vi "LWXPS_PositionerCompensationDualLoopNotchFilterGet.vi"(0 "XPS Reference IN":refnum<k24>, 5 "Positioner Name":string, 7 "Notch Number":i32, 11 "LabVIEW error IN":errorcluster) -> (3 "XPS Reference OUT":refnum<k24>, 4 "Returned error code":i32, 6 "Notch Frequency":dbl, 8 "Notch Bandwidth":dbl, 10 "Notch Gain":dbl, 14 "LabVIEW error OUT":errorcluster, 15 "XPS Error String":string)   [LabVIEW 2014]
uses:
  D:/XPSQ8_LabView_Library/Development/Source/Dll/Newport.XPS.CommandInterface.dll
  Dll/Newport.XPS.CommandInterface.dll
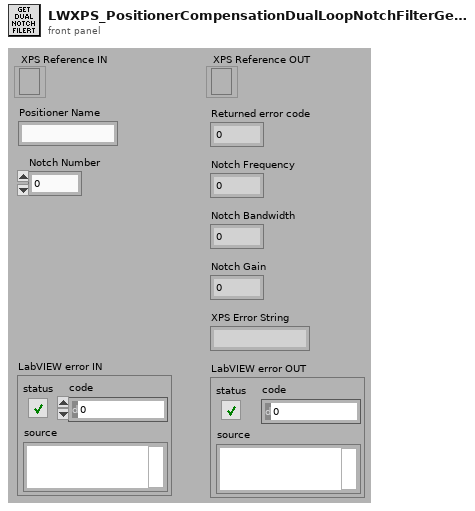
[diagram p1: front panel]
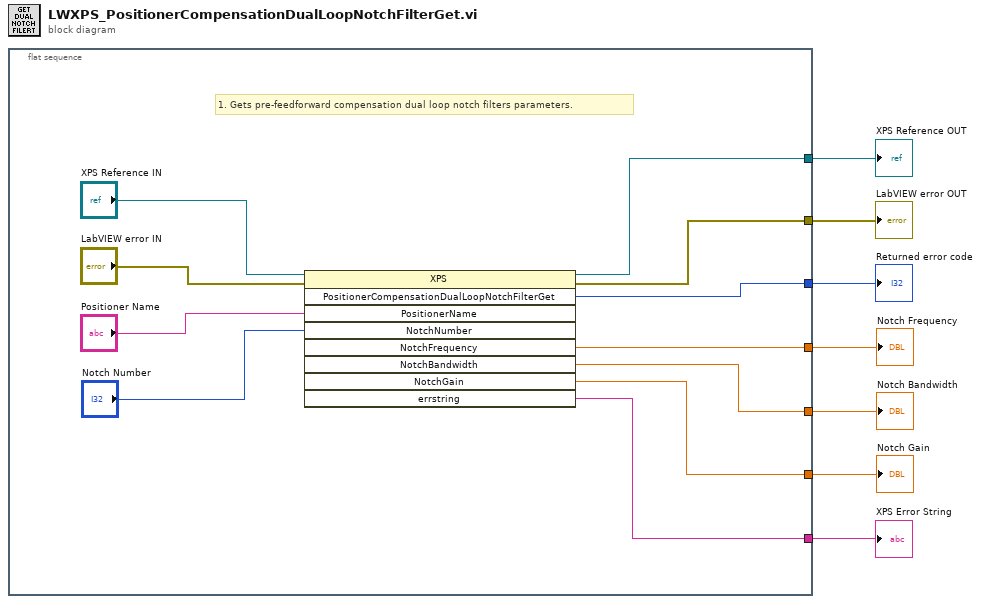
[diagram p0: block diagram]
diagram:
  n1 = flat-sequence {
    tunnel: [w17] -> w7
    tunnel: [w16] -> w6
    tunnel: [w15] -> w5
    tunnel: [w12] -> w4
    tunnel: [w8] -> w3
    tunnel: [w9] -> w2
    tunnel: [w11] -> w1
    frame #0 {
      # "1. Gets pre-feedforward compensation dual loop notch filters parameters."
      n2 = invoke class="XPS" method="PositionerCompensationDualLoopNotchFilterGet"(reference="XPS Reference IN", error in="LabVIEW error IN", "PositionerName"="Positioner Name", "NotchNumber"="Notch Number") -> (reference out=w17:refnum<k24>, error out=w16:errorcluster, "PositionerCompensationDualLoopNotchFilterGet"=w15:i32, "NotchFrequency"=w12:dbl, "NotchBandwidth"=w8:dbl, "NotchGain"=w9:dbl, "errstring"=w11:string)  [unwired: 5 in, 2 out]
    }
  }
  "XPS Error String" <- w1
  "XPS Reference OUT" <- w7
  "LabVIEW error OUT" <- w6
  "Returned error code" <- w5
  "Notch Frequency" <- w4
  "Notch Bandwidth" <- w3
  "Notch Gain" <- w2
